vi "labview master mohamad.vi"() -> ()   [LabVIEW 2016]
uses:
  Control 1.ctl
  <vilib>/MakerHub/LINX/Public/Peripherals/Analog/Analog Read 1 Chan.vi
  <vilib>/MakerHub/LINX/Public/Peripherals/Digital/Digital Read 1 Chan.vi
  <vilib>/MakerHub/LINX/Public/Peripherals/Analog/Analog Read N Chans.vi
  <vilib>/MakerHub/LINX/Public/Peripherals/Digital/Digital Read N Chans.vi
  <vilib>/MakerHub/LINX/Private/Local IO/LinxAnalogRead.vi
  <vilib>/MakerHub/LINX/Public/Utilities/Check Channel.vi
  <vilib>/MakerHub/LINX/Private/Local IO/LinxDigitalRead.vi
  <vilib>/MakerHub/LINX/Public/Utilities/Open Serial.vi
  <vilib>/MakerHub/LINX/Private/Utilties/Generate Error.vi
  <vilib>/MakerHub/LINX/LMH-LINX.lvlib
panel:
  out "حالة \nالطور الثالث":bool
  out "حالة\nالطور الثاني":bool
  out "حالة\nالطور الأول":bool
  in  "حالة الطور الثالث":u8
  in  "حالة الطور الأول":u8
  in  "حالة الطور الثاني":u8
  out "2":string
  out "الطور الأول":bool
  out "الطور الثاني":bool
  out "الطور الثالث":bool
  in  "الطور":u32(slide) scale=0.0..2.0
  out "ترتيب الأطوار":bool
  in  "ترتيب الاطوار":u8
  in  "DI Channel":u8
  out "Numeric Indicator":dbl
  out "Thermometer":dbl(slide) scale=0.0..100.0
  out "لمبة التهييج":bool
  out "انخفاض التردد":bool
  out "ارتفاع التردد":bool
  out "مقياس التردد":dbl(knob) scale=0.0..55.0
  in  "مدخل الحرارة":u8
  out "?":bool
  out "ارتفاع الجهد":bool
  in  "مدخل النردد":u8
  out "Boolean 2":bool
  in  "Boolean":bool
  in  "حالة الأطوار":u8
  out "حرارة \nتبريد المولد":bool
  out "مقياس الجهد الطور 1":T1 caption="مقياس الجهد" scale=0.0..460.0
  in  "Stop Button":bool
  out "Loop Rate (Hz)":u32
  in  "مدخل الجهد":u8
  in  "Serial Port":refnum<visa-resource-name>="N/A"
  # "انخفاض الجهد"
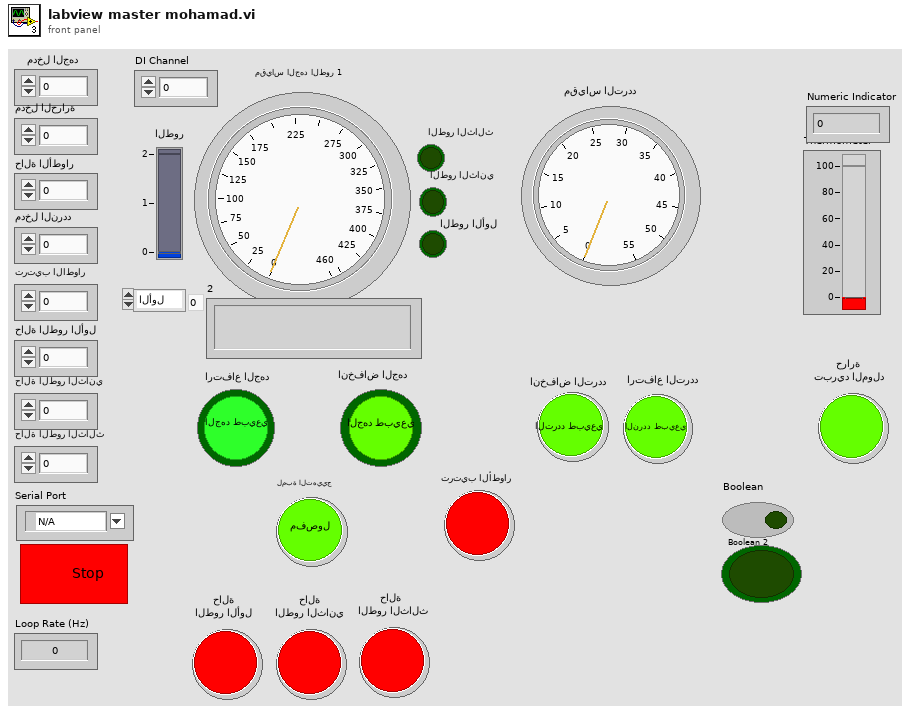
[diagram p1: front panel]
types:
  T1 = typedef "Control 1.ctl" = dbl
  T2 = typedef "LMH-LINX.lvlib/LINX Ref.ctl" = cluster{"IO":T3, "Interface":T4, "LINX Device Config":T5}
  T3 = typedef "LMH-LINX.lvlib/Platform.ctl" = enum16{"Remote", "Local"}
  T4 = typedef "LMH-LINX.lvlib/Interface.ctl" = enum16{"Serial", "TCP"}
  T5 = typedef "LMH-LINX.lvlib/Device.lvlib/LINX Device Config.ctl" = cluster{"Interface":T4, "COM Port":refnum<visa-resource-name>, "TCP Configuration":T6, "Device Family":u8, "Device ID":u8, "Device Name":string, "TCP Ref":refnum<k5>, "Channels":T7}
  T6 = typedef "LMH-LINX.lvlib/Device.lvlib/TCP Config.ctl" = cluster{"IP Address":string, "Port":u16}
  T7 = typedef "LMH-LINX.lvlib/Channels.ctl" = cluster{"DI":u8[], "DO":u8[], "AI":u8[], "AO":u8[], "PWM":u8[], "QE":u8[], "UART":u8[], "I2C 2":u8[], "SPI":u8[], "CAN":u8[], "Servo":u8[], "AI Ref (V)":dbl, "AI Resolution (Bits)":u8, "AO Ref (V)":dbl, "AO Resolution (Bits)":u8}
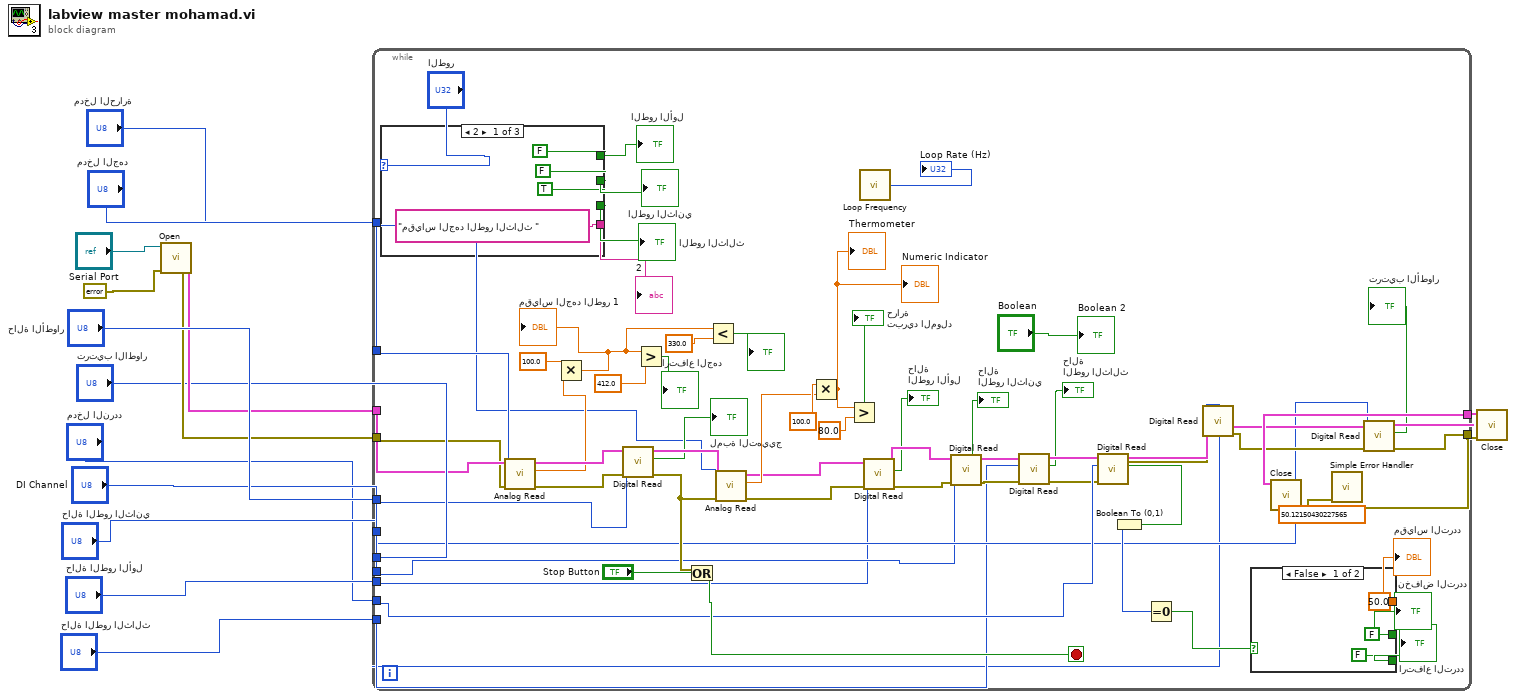
[diagram p0: block diagram]
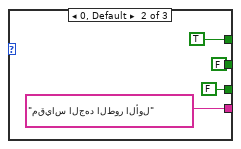
[diagram p2: hidden frame]
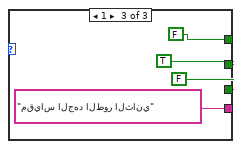
[diagram p3: hidden frame]
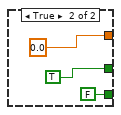
[diagram p4: hidden frame]
diagram:
  n1 = call-poly <vilib>:"Open.vi"("Error In"=errorcluster {"status"=FALSE, "code"=0, "source"=""}, "Serial Port"="Serial Port") -> ("Error Out"=w9:errorcluster, "LINX Resource"=w10:T2)  [unwired: 7 in, 1 out]
  n2 = while {
    tunnel: "مدخل الجهد" -> [w20]
    tunnel: "حالة الأطوار" -> [w18]
    tunnel: "مدخل النردد" -> [w57]
    tunnel: "مدخل الحرارة" -> [w19]
    tunnel: [w44] -> w3
    tunnel: w10 -> [w54]
    tunnel: w9 -> [w53]
    tunnel: "DI Channel" -> [w17]
    tunnel: [w43] -> w2
    tunnel: "ترتيب الاطوار" -> [w42]
    tunnel: "حالة الطور الثاني" -> [w26]
    tunnel: "حالة الطور الأول" -> [w25]
    tunnel: "حالة الطور الثالث" -> [w24]
    stop <- w75 stop-if-true
    (unwired) 50.12150430227565 ("مقياس التردد")
    n3 = case shown="2" "الطور" {
      tunnel: [FALSE TRUE FALSE] -> w35
      tunnel: [FALSE FALSE TRUE] -> w38
      tunnel: [TRUE FALSE FALSE] -> w37
      tunnel: ["مقياس الجهد الطور الثالث " "مقياس الجهد الطور الأول" "مقياس الجهد الطور الثاني"] -> w36
      frame 2 {
      }
      frame 0, Default {
      }
      frame 1 {
      }
    }
    "الطور الثالث" <- w37
    "الطور الثاني" <- w38
    "الطور الأول" <- w35
    "2" <- w36
    n4 = call-poly <vilib>:"Analog Read.vi"("Error In"=w53, "Analog Channel"=w20, "LINX Resource"=w54) -> ("Error Out"=w72:errorcluster, "Voltage"=w65:dbl, "LINX Resource"=w73:T2)  [unwired: 5 in, 1 out]
    n5 = Multiply(x=w65, y=100.0) -> (x*y=w40:dbl)
    "مقياس الجهد الطور 1" <- w40
    n6 = call-poly <vilib>:"Digital Read.vi"("Error In"=w72, "DI Channel"=w18, "LINX Resource"=w73) -> ("Error Out"=w66:errorcluster, "DI Value"=→"لمبة التهييج":bool, "LINX Resource"=w67:T2)  [unwired: 6 in]
    n7 = Greater?(x=w40, y=412.0) -> (0:→"ارتفاع الجهد":bool)
    n8 = Or(x=w66, y="Stop Button") -> (x .or. y?=w75:bool)
    n9 = Less?(x=w40, y=330.0) -> (x < y?=→"?":bool)
    n10 = call-poly <vilib>:"Analog Read.vi"("Error In"=w66, "Analog Channel"=w19, "LINX Resource"=w67) -> ("Error Out"=w32:errorcluster, "Voltage"=w62:dbl, "LINX Resource"=w29:T2)  [unwired: 5 in, 1 out]
    n11 = Multiply(x=100.0 ("y"), y=w62) -> (x*y=w59:dbl)
    "Thermometer" <- w59
    "Numeric Indicator" <- w59
    n12 = Greater?(x=w59, y=80.0) -> (0:→"حرارة \nتبريد المولد":bool)
    n13 = call <vilib>:"Loop Frequency.vi"() -> ("Loop Rate (Hz)"=→"Loop Rate (Hz)":u32)
    n14 = call-poly <vilib>:"Digital Read.vi"("Error In"=w32, "DI Channel"=w25, "LINX Resource"=w29) -> ("Error Out"=w31:errorcluster, "DI Value"=→"حالة\nالطور الأول":bool, "LINX Resource"=w34:T2)  [unwired: 6 in]
    n15 = call-poly <vilib>:"Digital Read.vi"("Error In"=w31, "DI Channel"=w26, "LINX Resource"=w34) -> ("Error Out"=w30:errorcluster, "DI Value"=→"حالة\nالطور الثاني":bool, "LINX Resource"=w33:T2)  [unwired: 6 in]
    n16 = call-poly <vilib>:"Digital Read.vi"("Error In"=w30, "DI Channel"=w24, "LINX Resource"=w33) -> ("Error Out"=w27:errorcluster, "DI Value"=→"حالة \nالطور الثالث":bool, "LINX Resource"=w28:T2)  [unwired: 6 in]
    n17 = call-poly <vilib>:"Digital Read.vi"("Error In"=w27, "DI Channel"=w57, "LINX Resource"=w28) -> ("Error Out"=w55:errorcluster, "DI Value"=w52:bool, "LINX Resource"=w56:T2)  [unwired: 6 in]
    n18 = Boolean To (0,1)(Boolean=w52) -> (0, 1=w51:i16)
    n19 = Equal To 0?(x=w51) -> (x = 0?=w50:bool)
    n20 = call-poly <vilib>:"Digital Read.vi"("Error In"=w55, "DI Channel"=w17, "LINX Resource"=w56) -> ("Error Out"=w45:errorcluster, "LINX Resource"=w46:T2)  [unwired: 6 in, 1 out]
    n21 = case shown="False" w50 {
      tunnel: [50.0 ("مقياس التردد") 0.0 ("مقياس التردد")] -> w49
      tunnel: [FALSE ("انخفاض التردد") TRUE ("انخفاض التردد")] -> w48
      tunnel: [FALSE FALSE] -> w47
      frame False {
      }
      frame True {
      }
    }
    "مقياس التردد" <- w49
    "انخفاض التردد" <- w48
    "ارتفاع التردد" <- w47
    n22 = call-poly <vilib>:"Digital Read.vi"("Error In"=w45, "DI Channel"=w42, "LINX Resource"=w46) -> ("Error Out"=w43:errorcluster, "DI Value"=→"ترتيب الأطوار":bool, "LINX Resource"=w44:T2)  [unwired: 6 in]
    "Boolean 2" <- "Boolean"
  }
  n23 = call <vilib>:"Close.vi"("Error In"=w2, "LINX Resource"=w3) -> ("Error Out"=w13:errorcluster)  [unwired: 9 in]
  n24 = call <vilib>:"Simple Error Handler.vi"("error in (no error)"=w13) -> ()  [unwired: 4 in, 5 out]
  n25 = call <vilib>:"Close.vi"("Error In"=w2, "LINX Resource"=w3) -> ()  [unwired: 9 in, 1 out]
